vi "Read Data Titles.vi"(8 "error in (no error)":errorcluster, 11 "EGG7260 in":refnum<class "EGG7260.lvclass">) -> (0 "error out":errorcluster, 2 "Data titles":string[](array[string])=["EGG7260_Vx (V)", "EGG7260_Vy (V)"], 3 "EGG7260 out":refnum<class "EGG7260.lvclass">)   [LabVIEW 2015, in "EGG7260.lvclass"]
uses:
  EGG7260.lvclass
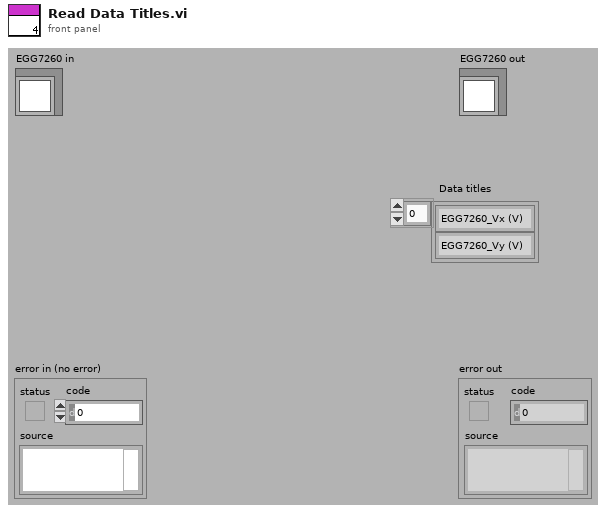
[diagram p1: front panel]
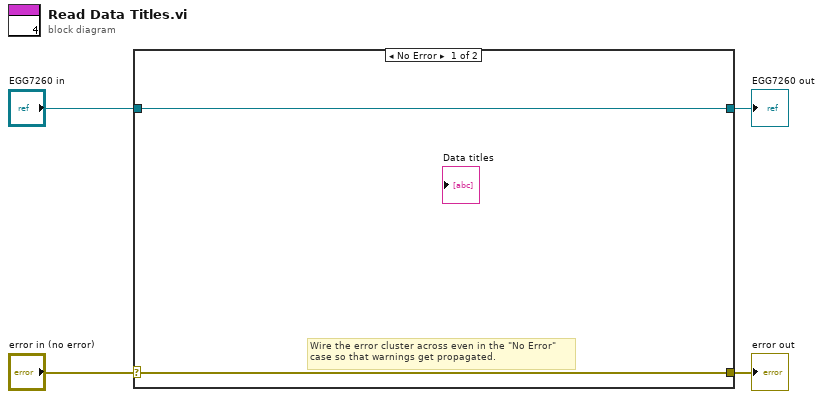
[diagram p0: block diagram]
diagram:
  n1 = case shown="No Error" "error in (no error)" {
    selector: "error in (no error)" -> [w5 w8]
    tunnel: [w5 w8] -> w3
    tunnel: [w6 w7] -> w1
    tunnel: "EGG7260 in" -> [w6 w7]
    frame No Error {
      # "Wire the error cluster across even in the \"No Error\"\ncase so that warnings get propagated."
    }
    frame Error {
    }
  }
  "error out" <- w3
  "EGG7260 out" <- w1
